vi "savedat1.vi"(2 "Array":cluster{"x0":dbl, "dx":dbl, "y":sgl[][]}[](array[cluster]), 4 "Time Stamp":timestamp) -> (0 "offset":i32)   [LabVIEW 2010]
uses:
  70user.lib/TheSigTab.vi
panel:
  in  "Case Constant\n(See Context Help)":bool=TRUE
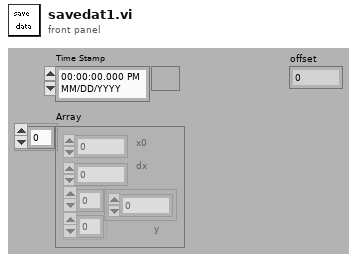
[diagram p1: front panel]
types:
  T1 = enum16{"open", "replace", "create", "open or create", "replace or create", "replace or create with confirmation"}
  T2 = cluster{"Time Stamp":timestamp, "Array":cluster{"x0":dbl, "dx":dbl, "y":sgl[][]}[]}
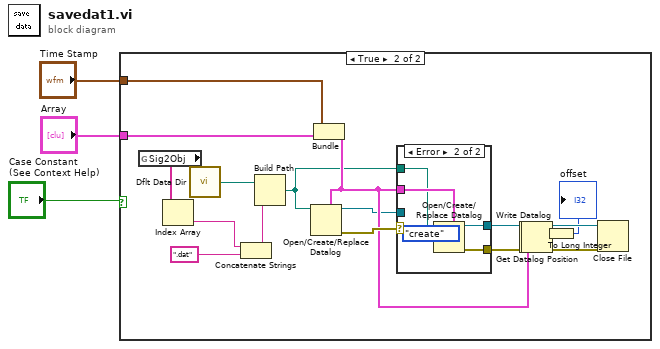
[diagram p0: block diagram]
diagram:
  n1 = case shown="True" "Case Constant\n(See Context Help)" {
    tunnel: "Time Stamp" -> [_ w18]
    tunnel: "Array" -> [_ w17]
    frame False {
    }
    frame True {
      n2 = global read "TheSigTab.vi" "Sig2Obj"() -> (w8:string[])
      n3 = Index Array(array=w8) -> (element=w7:string)  [unwired: 1 in]
      n4 = call <vilib>:"Dflt Data Dir.vi"() -> ("App:Default Data Directory"=w16:path)
      n5 = Concatenate Strings(w7, ".dat") -> (w14:string)
      n6 = Build Path(base path=w16, name or relative path=w14) -> (appended path=w10:path)
      n7 = Bundle("Time Stamp"=w18, "Array"=w17) -> (w12:T2)  [unwired: 1 in]
      n8 = Open/Create/Replace Datalog(5:w12, 11:w10) -> (0:w13:errorcluster, 3:w11:refnum<k1>)  [unwired: 4 in, 1 out]
      n9 = case shown="Error" w13 {
        selector: w13 -> [w23 _]
        tunnel: w12 -> [_ w27]
        tunnel: [w24 w29] -> w20
        tunnel: [w23 w28] -> w19
        tunnel: w11 -> [w24 _]
        tunnel: w10 -> [_ w26]
        frame No Error {
        }
        frame Error {
          n10 = Open/Create/Replace Datalog(5:w27, 10:T1."create" ("operation (0:open)"), 11:w26) -> (0:w28:errorcluster, 3:w29:refnum<k1>)  [unwired: 3 in, 1 out]
        }
      }
      n11 = Write Datalog(4:w19, 6:w12, 7:w20) -> (0:w5:errorcluster, 3:w6:refnum<k1>)
      n12 = Get Datalog Position(4:w5, 7:w6) -> (0:w21:errorcluster, 2:w4:i64, 3:w22:refnum<k1>)
      n13 = To Long Integer(number=w4) -> (32bit integer=→"offset":i32)
      n14 = Close File(refnum=w22, error in=w21) -> ()  [unwired: 2 out]
    }
  }
